vi "niRFUtil WFM Moving Average.vi"   [LabVIEW 2015, in "niRFUtil.lvlib"]
uses:
  niRFUtil.lvlib
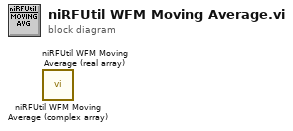
[diagram p0: block diagram]
diagram:
  n1 = call "niRFUtil WFM Moving Average (complex array).vi"() -> ()  [unwired: 15 in, 1 out]
  n2 = call "niRFUtil WFM Moving Average (real array).vi"() -> ()  [unwired: 15 in, 1 out]
